vi "Send Horizontal Settings.vi"(8 "error in":errorcluster, 11 "5105 in":refnum<class "5105.lvclass">) -> (0 "error out":errorcluster, 3 "5105 out":refnum<class "5105.lvclass">)   [LabVIEW 2019, in "5105.lvlib" / "5105.lvclass"]
uses:
  5105.lvclass
  C:/Users/Public/Documents/Development/builds/Instruments/Oscilloscope.lvlibp/Oscilloscope.lvclass
  Accessors/Read Local Resource.vi
  builds/Instruments/Oscilloscope.lvlibp/Accessors/Read Horizontal Setting.vi
  Accessors/Write Local Resource.vi
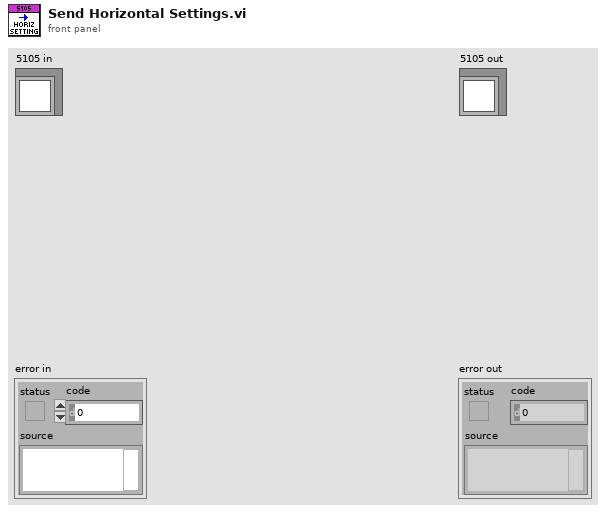
[diagram p1: front panel]
types:
  T1 = typedef "Oscilloscope.lvlibp/Oscilloscope.lvclass/Horizontal Setting.ctl" = cluster{"Num Records":i32, "Sample Rate":dbl, "Reference Pos":dbl, "Min Record len":i32}
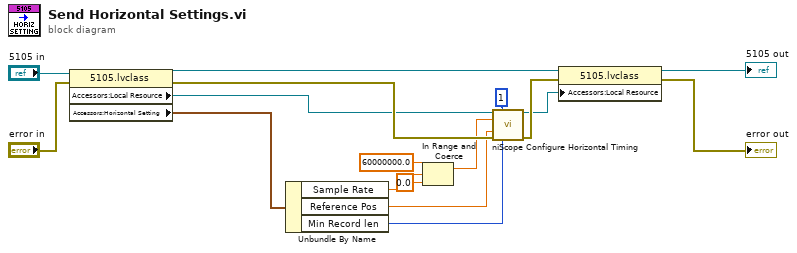
[diagram p0: block diagram]
diagram:
  n1 = property class="5105.lvclass"(reference="5105 in", error in="error in") -> (reference out=w15:refnum<class "5105.lvclass">, error out=w12:errorcluster, "Accessors:Local Resource"=w10:refnum<k15>, "Accessors:Horizontal Setting"=w11:T1)
  n2 = Unbundle By Name(w11) -> ("Sample Rate"=w4:dbl, "Reference Pos"=w8:dbl, "Min Record len"=w9:i32)
  n3 = In Range and Coerce(upper limit=60000000.0, x=w4, lower limit=0.0) -> (coerced(x)=w3:dbl)  [unwired: 1 out]
  n4 = call <instrlib>:"niScope Configure Horizontal Timing.vi"("instrument handle"=w10, "number of records"=1, "min sample rate"=w3, "reference position"=w8, "error in"=w12, "min record length"=w9) -> ("instrument handle out"=w6:refnum<k15>, "error out"=w7:errorcluster)  [unwired: 8 in]
  n5 = property class="5105.lvclass"(reference=w15, error in=w7, "Accessors:Local Resource"=w6) -> (reference out=→"5105 out":refnum<class "5105.lvclass">, error out=→"error out":errorcluster)
